vi "Main.vi"() -> ()   [LabVIEW 2012]
uses:
  Lucid/LabVIEW/dependencies/libraries/TIFFManagement_x32/TIFFManagement.lvlib
panel:
  out "x/y":dbl
  out "appended path":path
  out "Progress":dbl(slide) scale=0.0..100.0
  out "error out":errorcluster
  out "wrong files":path[](array[path])
  out "wrong folders":path[](array[path])
  in  "# of pages in 3D tiffs":i32
  in  "# of files in second level folders":i32
  in  "# of second level folders":i32
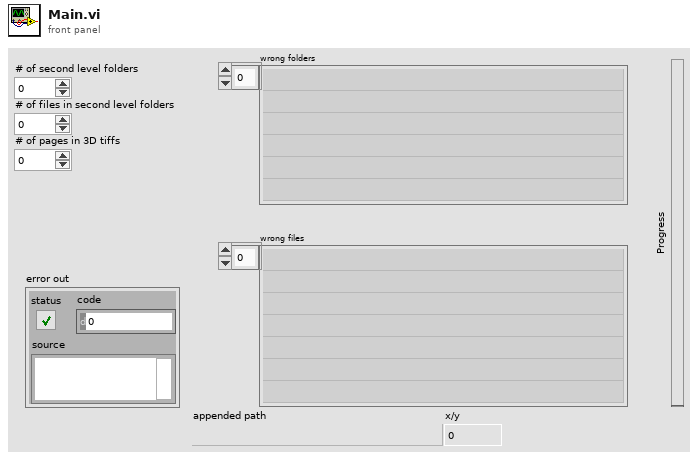
[diagram p1: front panel]
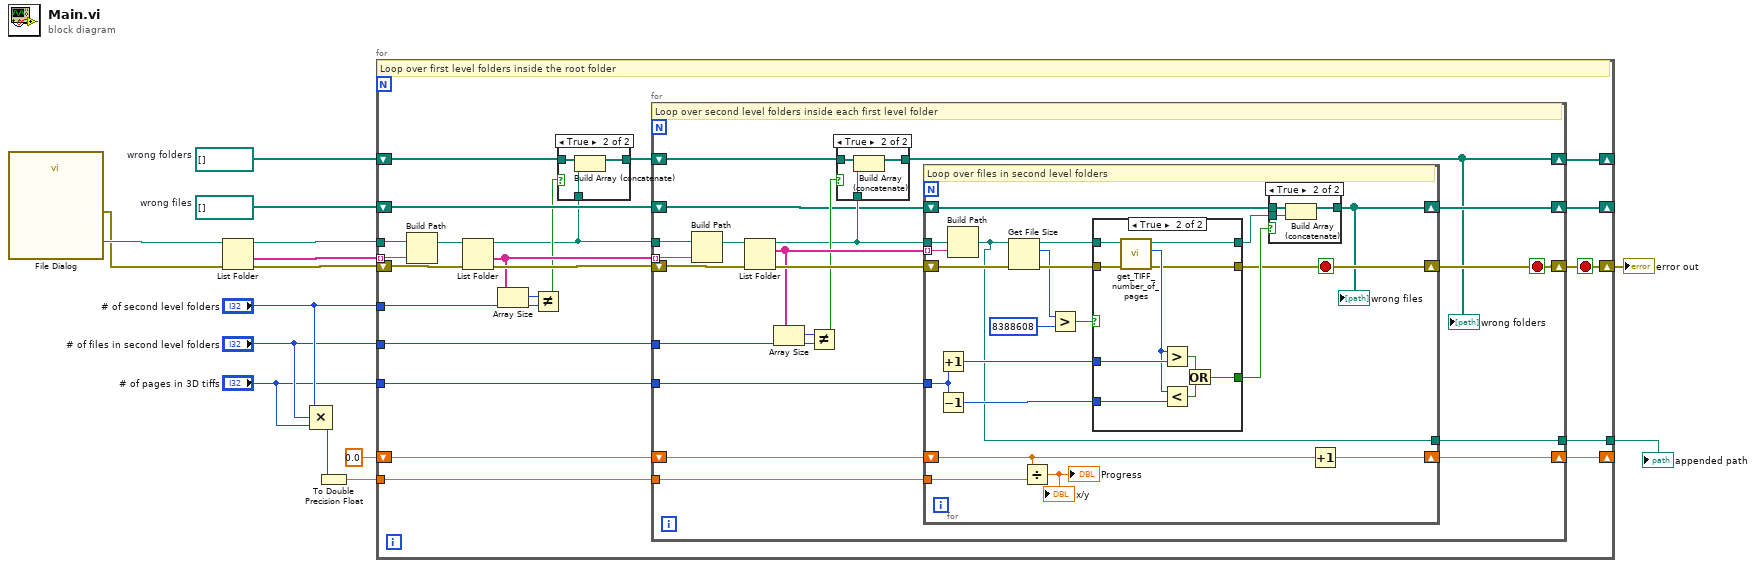
[diagram p0: block diagram]
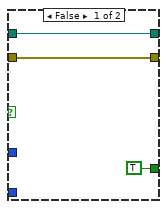
[diagram p4: hidden frame]
diagram:
  w11 = path[] []  # wrong files
  w12 = path[] []  # wrong folders
  n1 = call "File Dialog"() -> ("selected path"=w9:path, "error out"=w8:errorcluster)  [unwired: 12 in, 2 out]
  n2 = List Folder ("root folder")(path=w9, error in=w8) -> (path out=w13:path, folder names=w15:string[], error out=w14:errorcluster)  [unwired: 2 in, 1 out]
  n3 = Compound Arithmetic op=MULTIPLY("# of second level folders", "# of files in second level folders", "# of pages in 3D tiffs") -> (w3:i32)
  n4 = To Double Precision Float(number=w3) -> (double precision float=w2:dbl)
  n5 = for {
    tunnel: w15 -> [w36] mode=indexing
    shift-right: [w20] -> w10
    shift-left: w14 -> [w35]
    tunnel: w13 -> [w37]
    shift-right: [w23] -> _
    shift-left: w12 -> [w28]
    shift-right: [w21] -> _
    shift-left: w11 -> [w32]
    tunnel: "# of second level folders" -> [w29]
    tunnel: "# of files in second level folders" -> [w24]
    tunnel: "# of pages in 3D tiffs" -> [w22]
    shift-right: [w18] -> _
    shift-left: 0.0 ("# of pages in 3D tiffs") -> [w19]
    tunnel: w2 -> [w17]
    tunnel: [w16] -> w1
    stop <- w20 stop-if-true
    # "Loop over first level folders inside the root folder"
    n6 = Build Path(base path=w37, name or relative path=w36) -> (appended path=w34:path)
    n7 = List Folder(path=w34, error in=w35) -> (path out=w25:path, folder names=w31:string[], error out=w33:errorcluster)  [unwired: 2 in, 1 out]
    n8 = Array Size(array=w31) -> (size(s)=w30:i32)
    n9 = Not Equal?(x=w30, y=w29) -> (x != y?=w26:bool)
    n10 = case shown="True" w26 {
      tunnel: w28 -> [w38 w41]
      tunnel: [w38 w39] -> w27
      tunnel: w25 -> [_ w40]
      frame False {
      }
      frame True {
        n11 = Build Array (concatenate)(w41, w40) -> (w39:path[])
      }
    }
    n12 = for {
      tunnel: w25 -> [w61]
      tunnel: w31 -> [w60] mode=indexing
      shift-right: [w47] -> w20
      shift-left: w33 -> [w59]
      shift-right: [w43] -> w23
      shift-left: w27 -> [w53]
      shift-right: [w48] -> w21
      shift-left: w32 -> [w50]
      tunnel: w24 -> [w54]
      tunnel: w22 -> [w49]
      shift-right: [w45] -> w18
      shift-left: w19 -> [w46]
      tunnel: w17 -> [w44]
      tunnel: [w42] -> w16
      stop <- w47 stop-if-true
      # "Loop over second level folders inside each first level folder"
      n13 = Build Path(base path=w61, name or relative path=w60) -> (appended path=w58:path)
      n14 = List Folder(path=w58, error in=w59) -> (path out=w51:path, filenames=w55:string[], error out=w57:errorcluster)  [unwired: 2 in, 1 out]
      n15 = Array Size(array=w55) -> (size(s)=w56:i32)
      n16 = Not Equal?(x=w56, y=w54) -> (x != y?=w52:bool)
      n17 = case shown="True" w52 {
        tunnel: w53 -> [w62 w65]
        tunnel: [w62 w63] -> w43
        tunnel: w51 -> [_ w64]
        frame False {
        }
        frame True {
          n18 = Build Array (concatenate)(w65, w64) -> (w63:path[])
        }
      }
      "wrong folders" <- w43
      n19 = for {
        tunnel: w51 -> [w84]
        tunnel: w55 -> [w85] mode=indexing
        shift-right: [w67] -> w48
        shift-left: w50 -> [w80]
        shift-right: [w77] -> w47
        shift-left: w57 -> [w76]
        tunnel: w49 -> [w83]
        shift-right: [w71] -> w45
        shift-left: w46 -> [w69]
        tunnel: w44 -> [w70]
        tunnel: [w66] -> w42
        stop <- w77 stop-if-true
        # "Loop over files in second level folders"
        n20 = Increment(x=w83) -> (x+1=w82:i32)
        n21 = Decrement(x=w83) -> (x-1=w81:i32)
        n22 = Build Path(base path=w84, name or relative path=w85) -> (appended path=w66:path)
        n23 = Get File Size(file=w66, error in=w76) -> (size (in bytes)=w73:i64, 0:w75:errorcluster)  [unwired: 1 out]
        n24 = Divide(x=w69, y=w70) -> (x/y=→"Progress" →"x/y":dbl)
        n25 = Greater?(x=w73, y=i64 8388608) -> (0:w74:bool)
        n26 = case shown="True" w74 {
          tunnel: w82 -> [_ w98]
          tunnel: w81 -> [_ w97]
          tunnel: [w87 w93] -> w79
          tunnel: [TRUE w92] -> w78
          tunnel: [w88 w91] -> w77
          tunnel: w75 -> [w88 w90]
          tunnel: w66 -> [w87 w89]
          frame False {
          }
          frame True {
            n27 = call "get_TIFF_number_of_pages.vi"("error in (no error)"=w90, "path in"=w89) -> ("error out"=w91:errorcluster, "number of pages"=w96:i32, "path out"=w93:path)  [unwired: 7 in]
            n28 = Greater?(x=w96, y=w98) -> (0:w94:bool)
            n29 = Less?(x=w96, y=w97) -> (x < y?=w95:bool)
            n30 = Or(x=w94, y=w95) -> (x .or. y?=w92:bool)
          }
        }
        n31 = case shown="True" w78 {
          tunnel: w80 -> [w99 w102]
          tunnel: [w99 w100] -> w67
          tunnel: w79 -> [_ w101]
          frame False {
          }
          frame True {
            n32 = Build Array (concatenate)(w102, w101) -> (w100:path[])
          }
        }
        "wrong files" <- w67
        n33 = Increment(x=w69) -> (x+1=w71:dbl)
      }
    }
  }
  "error out" <- w10
  "appended path" <- w1
